vi "ExperimentLogLoop.vi"(8 "Error In":errorcluster, 9 "ABLE Configuration":T1, 10 "Experiment Log Data":refnum<queue>, 11 "Experiment Log Action Queue":refnum<queue>) -> (0 "Error Out":errorcluster)   [LabVIEW 2012]
uses:
  ABLEConfiguration.ctl
  DisplayConfiguration.ctl
  FolderConfiguration.ctl
  AlarmsConfiguration.ctl
  Keithley6485Configuration.ctl
  Keithley6482Configuration.ctl
  ExperimentLogActionQueueElement.ctl
  ExperimentLogAction.ctl
  ExperimentLogData.ctl
  ExperimentData.ctl
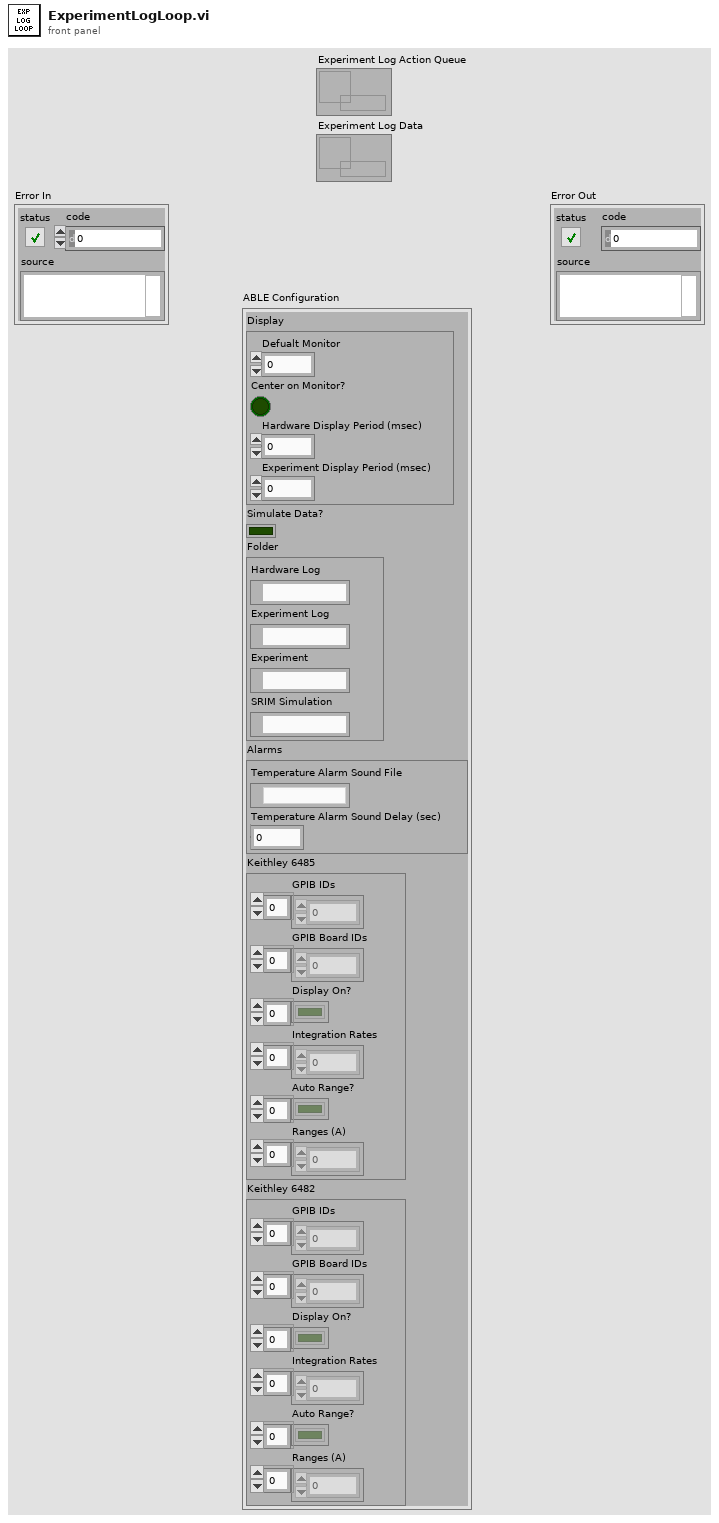
[diagram p1: front panel]
types:
  T1 = typedef "ABLEConfiguration.ctl" = cluster{"Display":T2, "Simulate Data?":bool, "Folder":T3, "Alarms":T4, "Keithley 6485":T5, "Keithley 6482":T6}
  T2 = typedef "DisplayConfiguration.ctl" = cluster{"Defualt Monitor":u16, "Center on Monitor?":bool, "Hardware Display Period (msec)":u32, "Experiment Display Period (msec)":u32}
  T3 = typedef "FolderConfiguration.ctl" = cluster{"Hardware Log":path, "Experiment Log":path, "Experiment":path, "SRIM Simulation":path}
  T4 = typedef "AlarmsConfiguration.ctl" = cluster{"Temperature Alarm Sound File":path, "Temperature Alarm Sound Delay (sec)":dbl}
  T5 = typedef "Keithley6485Configuration.ctl" = cluster{"GPIB IDs":u8[], "GPIB Board IDs":u8[], "Display On?":bool[], "Integration Rates":dbl[], "Auto Range?":bool[], "Ranges (A)":dbl[]}
  T6 = typedef "Keithley6482Configuration.ctl" = cluster{"GPIB IDs":u8[], "GPIB Board IDs":u8[], "Display On?":bool[], "Integration Rates":dbl[], "Auto Range?":bool[], "Ranges (A)":dbl[]}
  T7 = typedef "ExperimentLogActionQueueElement.ctl" = cluster{"Action":T8, "Data":variant}
  T8 = typedef "ExperimentLogAction.ctl" = enum16{"Initialize", "Clear", "Create", "Log", "Stop", "Shutdown"}
  T9 = enum16{"open", "replace", "create", "open or create", "replace or create", "replace or create with confirmation"}
  T10 = typedef "ExperimentLogData.ctl" = cluster{"Time Stamp":timestamp, "Experiment Data":T11}
  T11 = typedef "ExperimentData.ctl" = cluster{"Flux (ions/s * cm^2)":dbl, "Average Flux (ions/s * cm^2)":dbl, "DPA Rate":dbl, "Average DPA Rate":dbl, "Total Ion Energy (MeV)":dbl, "Total Charge (C)":dbl, "Dose (DPA)":dbl, "Fluence (ions/cm^2)":dbl, "Percent Complete (%)":dbl, "Duration (sec)":dbl}
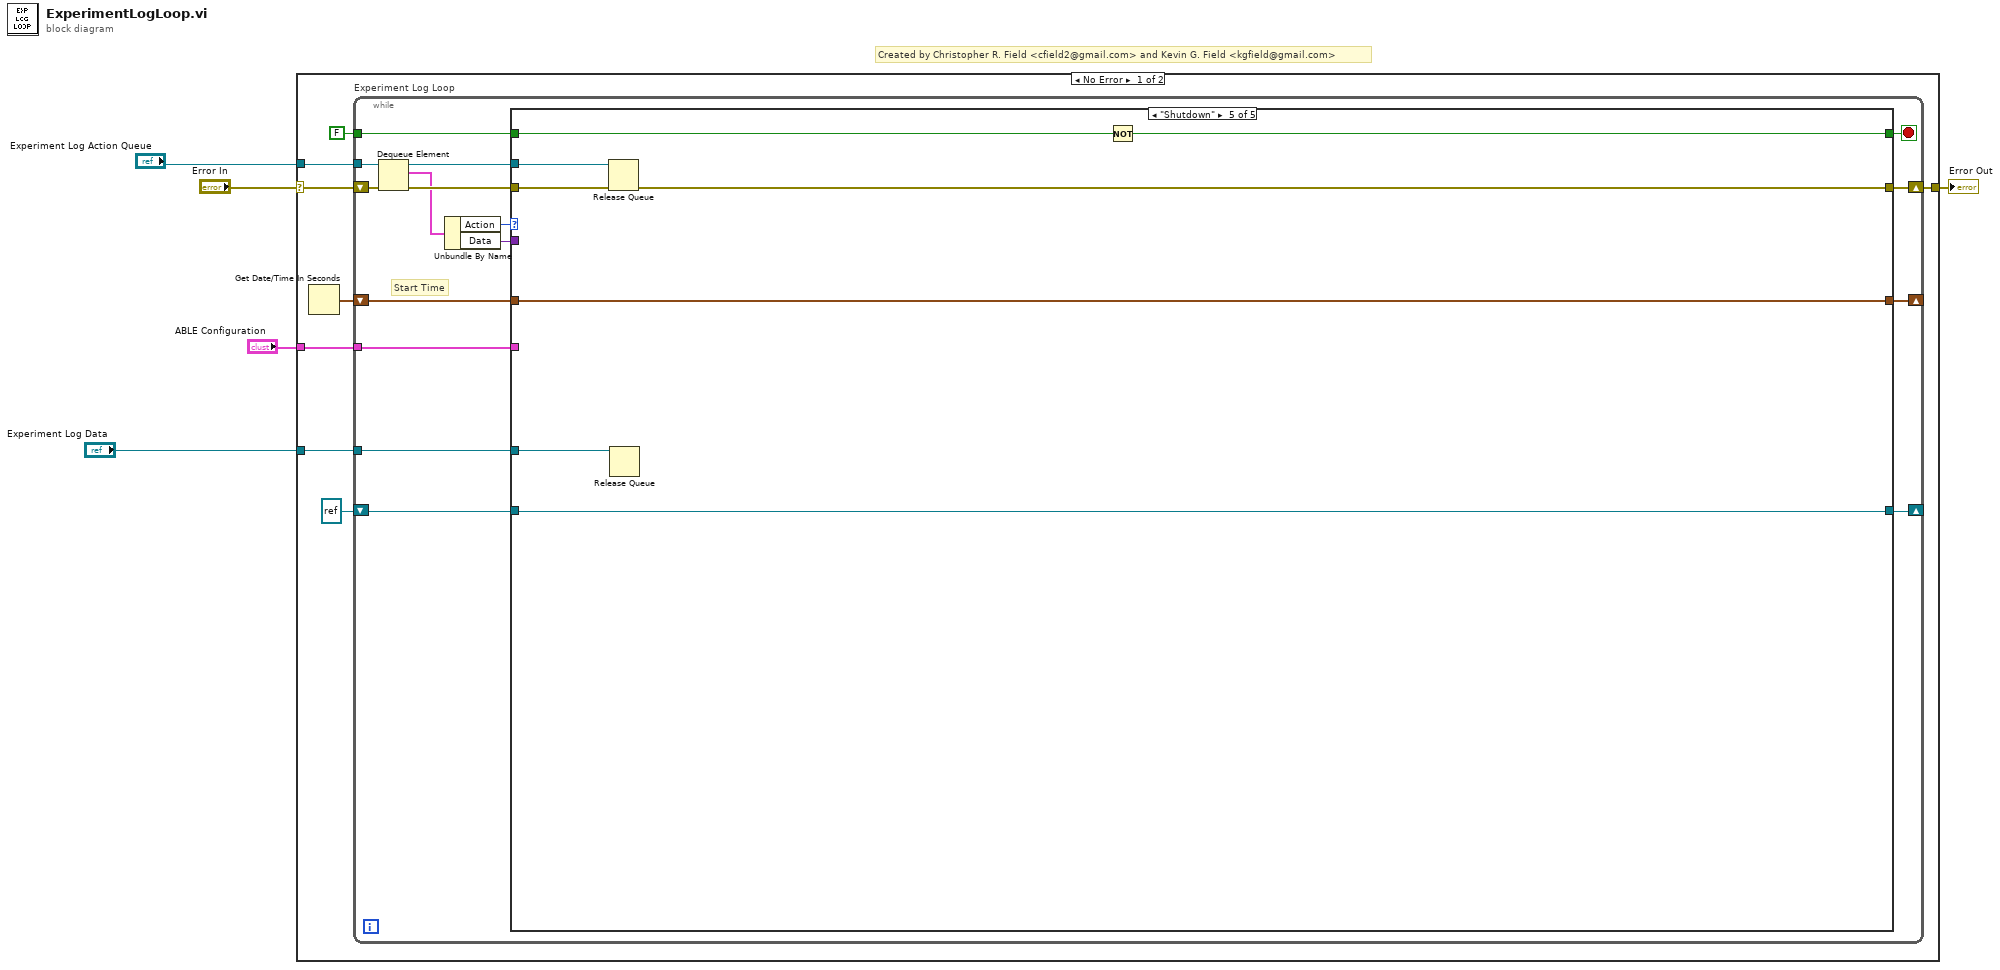
[diagram p0: block diagram]
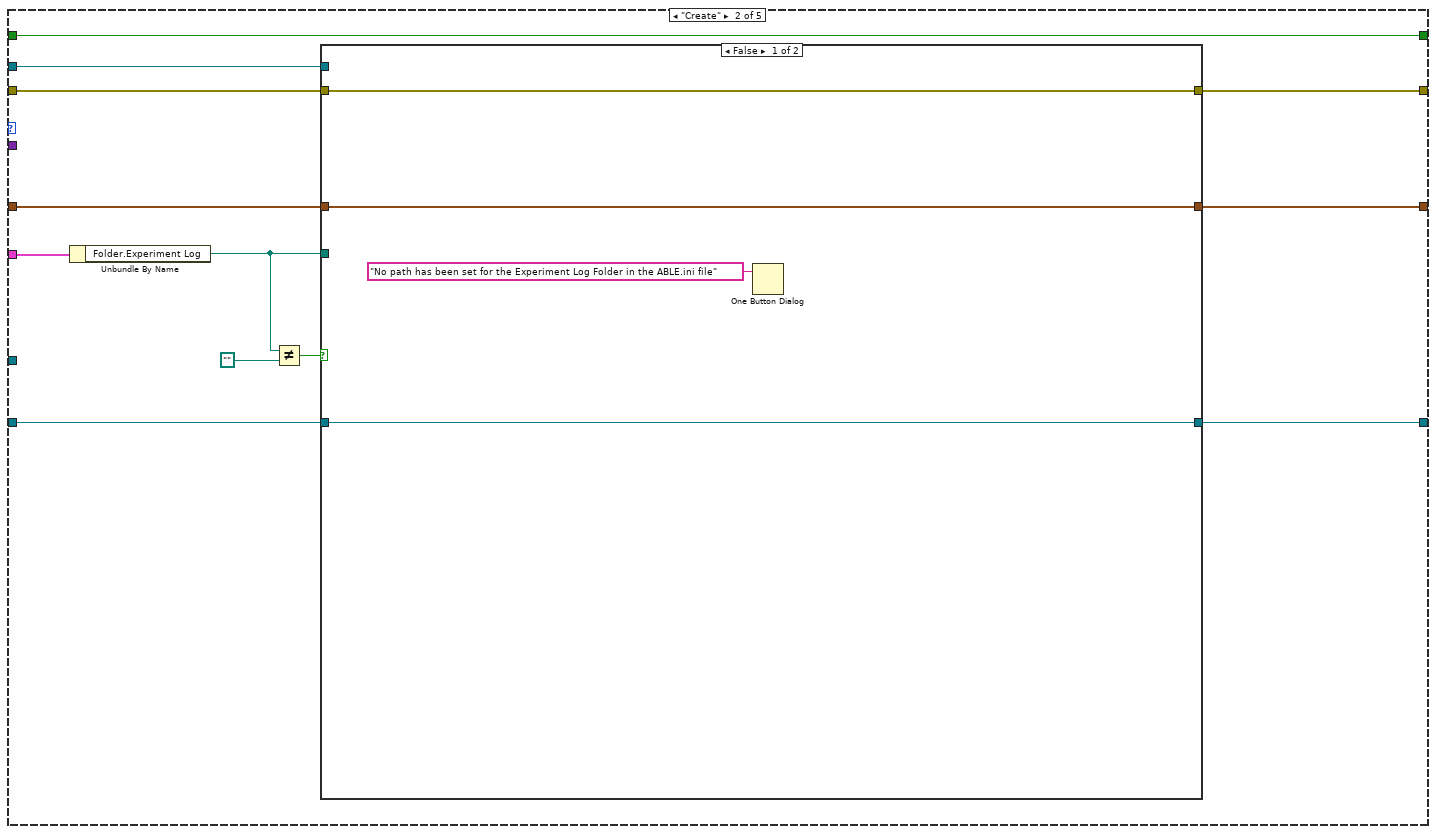
[diagram p3: hidden frame]
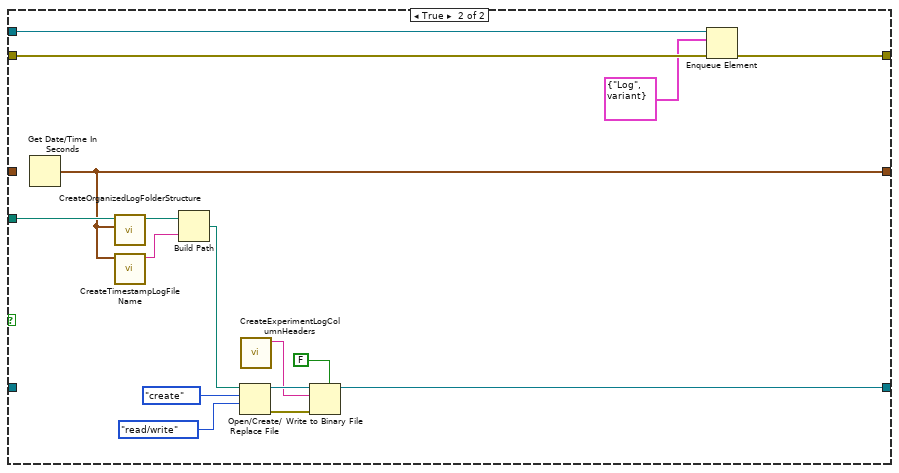
[diagram p4: hidden frame]
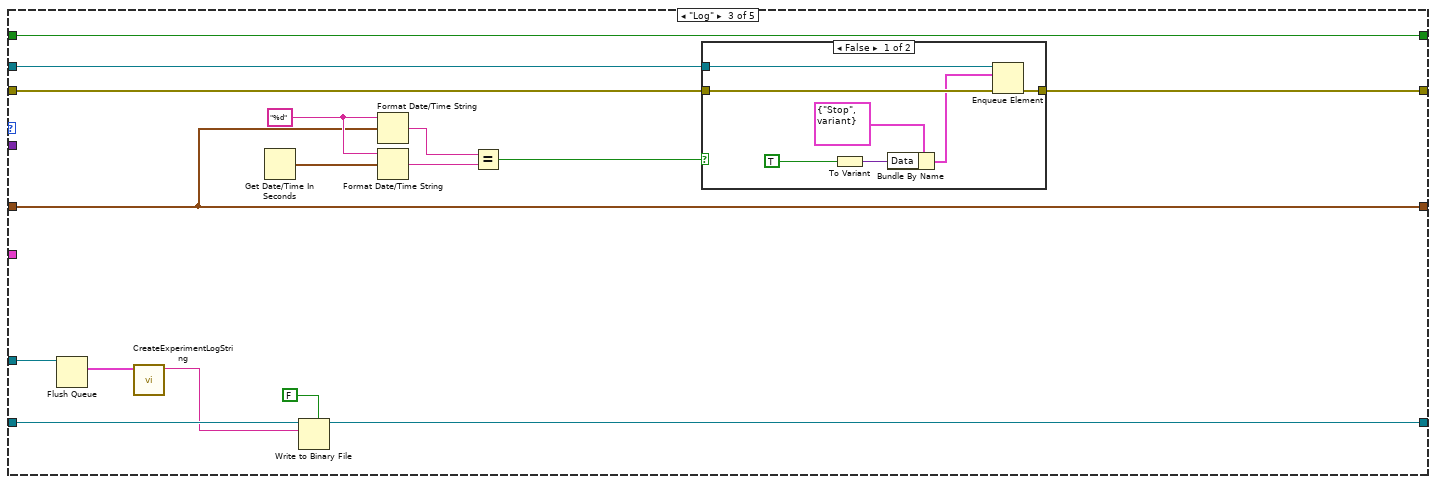
[diagram p5: hidden frame]
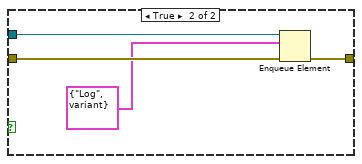
[diagram p6: hidden frame]
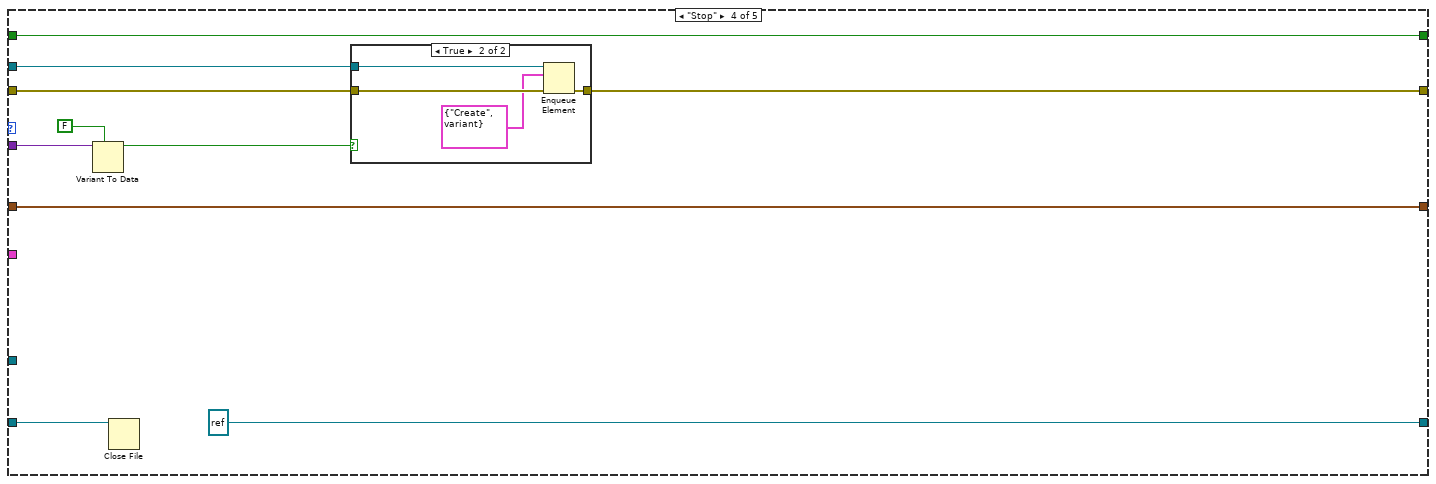
[diagram p7: hidden frame]
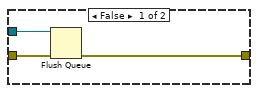
[diagram p8: hidden frame]
diagram:
  # "Created by Christopher R. Field <cfield2@gmail.com> and Kevin G. Field <kgfield@gmail.com>"
  n1 = case shown="No Error" "Error In" {
    selector: "Error In" -> [w12 w118]
    tunnel: [w11 w118] -> w5
    tunnel: "ABLE Configuration" -> [w8 _]
    tunnel: "Experiment Log Action Queue" -> [w10 _]
    tunnel: "Experiment Log Data" -> [w9 _]
    frame No Error {
      n2 = Get Date/Time In Seconds() -> (seconds since 1Jan1904=w6:timestamp)
      n3 = while "Experiment Log Loop" {
        tunnel: FALSE -> [w29]
        shift-right: [w26] -> w11
        shift-left: w12 -> [w28]
        tunnel: w10 -> [w20]
        tunnel: w9 -> [w19]
        tunnel: w8 -> [w18]
        shift-right: [w17] -> _
        shift-left: refnum<file> refnum ("refnum out") -> [w16]
        shift-right: [w15] -> _
        shift-left: w6 -> [w14]
        stop <- w21 stop-if-true
        # "Start Time"
        n4 = Dequeue Element(queue=w20, error in (no error)=w28) -> (queue out=w22:refnum<queue>, element=w25:T7, error out=w27:errorcluster)  [unwired: 1 in, 1 out]
        n5 = Unbundle By Name(w25) -> ("Action"=w24:T8, "Data"=w23:variant)
        n6 = case shown="\"Shutdown\"" w24 {
          tunnel: w29 -> [w33 w45 w81 w102 w117]
          tunnel: w27 -> [w30 w35 w79 w94 w113]
          tunnel: [w30 w34 w78 w93 w112] -> w26
          tunnel: w23 -> [_ _ _ w98 _]
          tunnel: w22 -> [_ w36 w80 w96 w114]
          tunnel: [w33 w45 w81 w102 w116] -> w21
          tunnel: w19 -> [_ _ w72 _ w115]
          tunnel: w18 -> [_ w44 _ _ _]
          tunnel: [w31 w40 w69 refnum<file> refnum ("refnum out") w110] -> w17
          tunnel: w16 -> [w31 w39 w71 w99 w110]
          tunnel: [w32 w38 w73 w101 w111] -> w15
          tunnel: w14 -> [w32 w37 w73 w101 w111]
          frame "Initialize", Default {
          }
          frame "Create" {
            n7 = Unbundle By Name(w44) -> ("Folder.Experiment Log"=w41:path)
            n8 = Not Equal?(x=w41, y=path "") -> (x != y?=w42:bool)
            n9 = case shown="False" w42 {
              tunnel: w41 -> [_ w58]
              tunnel: [w49 w60] -> w40
              tunnel: w39 -> [w49 _]
              tunnel: [w48 w56] -> w38
              tunnel: w37 -> [w48 _]
              tunnel: w36 -> [_ w54]
              tunnel: w35 -> [w47 w53]
              tunnel: [w47 w51] -> w34
              frame False {
                n10 = One Button Dialog(message="No path has been set for the Experiment Log Folder in the ABLE.ini file") -> ()  [unwired: 1 in, 1 out]
              }
              frame True {
                n11 = Get Date/Time In Seconds() -> (seconds since 1Jan1904=w56:timestamp)
                n12 = call "CreateOrganizedLogFolderStructure.vi"("Time Stamp"=w56, "Base Log Path"=w58) -> ("Organized Log Path"=w57:path)  [unwired: 8 in, 1 out]
                n13 = call "CreateTimestampLogFileName.vi"("Time Stamp"=w56) -> ("Timestamp Log File Name"=w55:string)  [unwired: 10 in]
                n14 = Build Path(base path=w57, name or relative path=w55) -> (appended path=w65:path)
                n15 = Open/Create/Replace File(file path (use dialog)=w65, operation (0:open)=T9."create", access (0:read/write)=enum16{"read/write", "read-only", "write-only"}."read/write") -> (refnum out=w62:refnum<file>, error out=w61:errorcluster)  [unwired: 3 in, 1 out]
                n16 = call "CreateExperimentLogColumnHeaders.vi"() -> ("Column Headers"=w50:string)  [unwired: 11 in]
                n17 = Write to Binary File(file (use dialog)=w62, data=w50, error in=w61, 5:FALSE ("prepend array or string size? (T)")) -> (refnum out=w60:refnum<file>)  [unwired: 2 in, 2 out]
                n18 = Enqueue Element(queue=w54, element=T7 {"Action"=enum."Log", "Data"=variant}, error in (no error)=w53) -> (error out=w51:errorcluster)  [unwired: 1 in, 2 out]
              }
            }
          }
          frame "Log" {
            w76 = "%d" ("time format string (%c)")
            n19 = Flush Queue(queue=w72) -> (remaining elements=w68:T10[])  [unwired: 1 in, 2 out]
            n20 = call "CreateExperimentLogString.vi"("Experiment Log Data Queue Elements"=w68) -> ("Experiment Log String"=w67:string)  [unwired: 10 in]
            n21 = Get Date/Time In Seconds() -> (seconds since 1Jan1904=w77:timestamp)
            n22 = Write to Binary File(file (use dialog)=w71, data=w67, 5:FALSE ("prepend array or string size? (T)")) -> (refnum out=w69:refnum<file>)  [unwired: 3 in, 2 out]
            n23 = Format Date/Time String(time format string (%c)=w76, seconds (now)=w73) -> (date/time string=w75:string)  [unwired: 1 in]
            n24 = Format Date/Time String(time format string (%c)=w76, seconds (now)=w77) -> (date/time string=w74:string)  [unwired: 1 in]
            n25 = Equal?(x=w75, y=w74) -> (x = y?=w66:bool)
            n26 = case shown="False" w66 {
              tunnel: w80 -> [w88 w92]
              tunnel: w79 -> [w87 w91]
              tunnel: [w86 w90] -> w78
              frame False {
                n27 = To Variant(anything=TRUE) -> (Variant=w84:variant)
                n28 = Bundle By Name(cluster=T7 {"Action"=enum."Stop", "Data"=variant} ("element"), "Data"=w84) -> (w82:T7)
                n29 = Enqueue Element(queue=w88, element=w82, error in (no error)=w87) -> (error out=w86:errorcluster)  [unwired: 1 in, 2 out]
              }
              frame True {
                n30 = Enqueue Element(queue=w92, element=T7 {"Action"=enum."Log", "Data"=variant}, error in (no error)=w91) -> (error out=w90:errorcluster)  [unwired: 1 in, 2 out]
              }
            }
          }
          frame "Stop" {
            n31 = Variant To Data(type=FALSE, Variant=w98) -> (data=w95:bool)  [unwired: 1 in, 1 out]
            n32 = Close File(refnum=w99) -> ()  [unwired: 1 in, 2 out]
            n33 = case shown="True" w95 {
              tunnel: w96 -> [w105 w109]
              tunnel: w94 -> [w104 w108]
              tunnel: [w103 w107] -> w93
              frame False {
                n34 = Flush Queue(queue=w105, error in (no error)=w104) -> (error out=w103:errorcluster)  [unwired: 2 out]
              }
              frame True {
                n35 = Enqueue Element(queue=w109, element=T7 {"Action"=enum."Create", "Data"=variant}, error in (no error)=w108) -> (error out=w107:errorcluster)  [unwired: 1 in, 2 out]
              }
            }
          }
          frame "Shutdown" {
            n36 = Release Queue(queue=w114, error in (no error)=w113) -> (error out=w112:errorcluster)  [unwired: 1 in, 2 out]
            n37 = Release Queue(queue=w115) -> ()  [unwired: 2 in, 3 out]
            n38 = Not(x=w117) -> (.not. x?=w116:bool)
          }
        }
      }
    }
    frame Error {
    }
  }
  "Error Out" <- w5
